vi "Get_PropID.vi"(11 "Prop":u16(ring) items=["AxTargetPosition"=44, "AxTargetVelocity"=45, "AxTargetTorque"=46, "AxControlWord"=47, "AxStatusWord"=48, "AxOperationMode"=49, "AxMaxTorque"=333]) -> (2 "BufferLength":u32, 3 "PropID":u32)   [LabVIEW 2020, in "输出轴伺服.lvlib"]
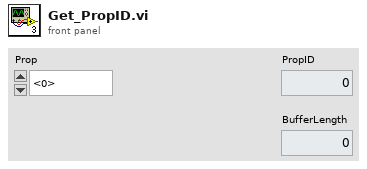
[diagram p1: front panel]
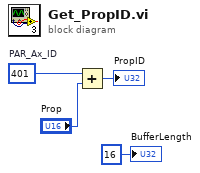
[diagram p0: block diagram]
diagram:
  w2 = 401  # PAR_Ax_ID
  n1 = Add(x=w2, y="Prop") -> (x+y=→"PropID":i32)
  "BufferLength" <- u32 16 ("BufferLength")
